vi "Test all.vi"   [LabVIEW 2018]
uses:
  <vilib>/addons/_JKI Toolkits/Caraya/classes/Test/Test.lvclass
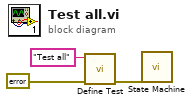
[diagram p0: block diagram]
diagram:
  n1 = call <vilib>:"Define Test.vi"("error in (no error)"=errorcluster {"status"=FALSE, "code"=0, "source"=""}, "Label (VI Title)"="Test all") -> ("error out"=w3:errorcluster)  [unwired: 8 in, 1 out]
  n2 = call "State Machine.vi"("error in (no error)"=w3) -> ()  [unwired: 10 in, 1 out]
